vi "test_MonoOpenAndInit.vi"(6 "Delay between send and receive [ms]":i32=100, 7 "Test should pass":bool=TRUE, 8 "error in":errorcluster, 9 "tear down connection":bool=TRUE, 10 "set-up a connection":bool=TRUE, 11 "device selection":enum16{"monochromator", "CCD", "SCD"}(ring)) -> (0 "error out":errorcluster, 1 "log-file path":path)   [LabVIEW 2023]
uses:
  Classes/Mono/Monochromator.lvclass
  <vilib>/addons/_JKI Toolkits/Caraya/classes/Assert/Assert Not Error.vi
  <vilib>/addons/_JKI Toolkits/Caraya/classes/Assert/Assert Equal Value and Type_Variant.vi
  <vilib>/addons/_JKI Toolkits/Caraya/classes/Test/Test.lvclass
  <vilib>/addons/_JKI Toolkits/Caraya/classes/Assert/Assert.lvclass
  <vilib>/Hampel Software Engineering/HSE Logger/hse-logger.lvlib
  C:/Users/grju/Desktop/AbgelegteDokumente/Kunden/Horiba/horiba-labview-sdk/Source/Classes/GenericDevice/GenericDevice.lvclass
  C:/Users/grju/Desktop/AbgelegteDokumente/Kunden/Horiba/horiba-labview-sdk/Source/Classes/Mono/Monochromator.lvclass
panel:
  in  "total time out [minutes]":i32=3
  # "Connector Pane"
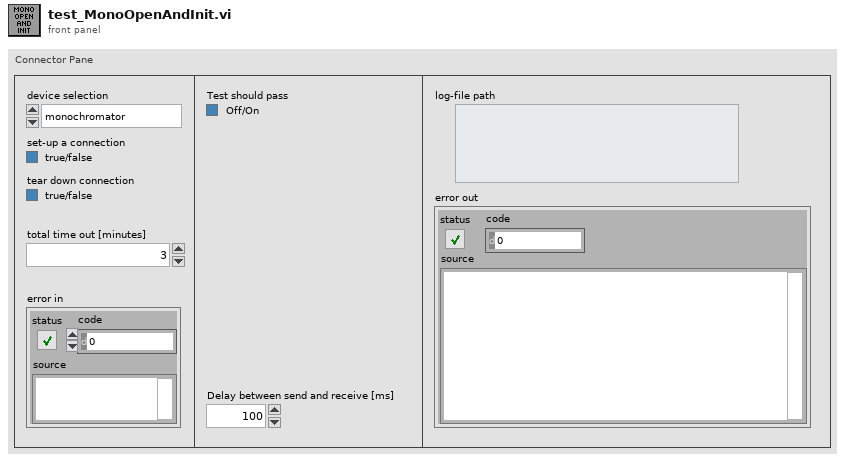
[diagram p1: front panel]
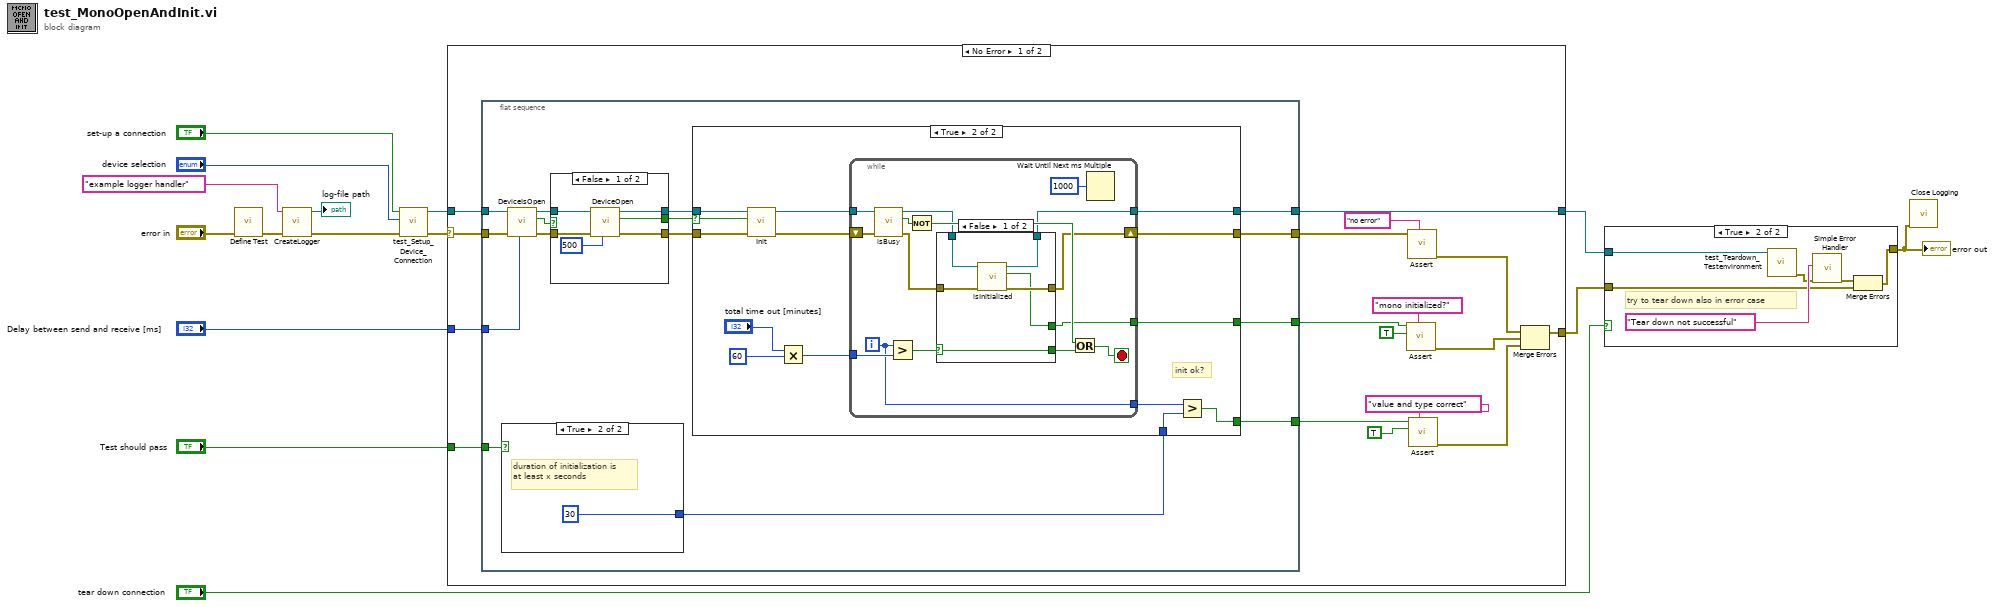
[diagram p0: block diagram]
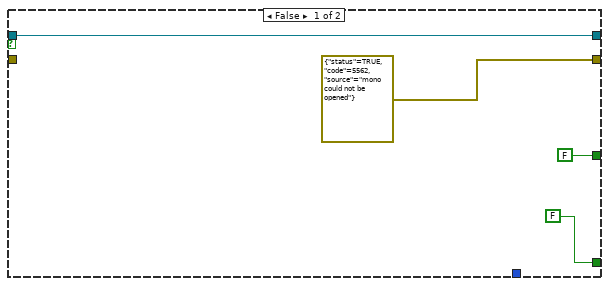
[diagram p2: hidden frame]
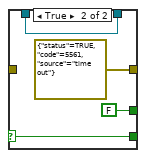
[diagram p3: hidden frame]
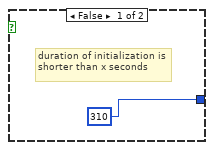
[diagram p5: hidden frame]
diagram:
  n1 = call <vilib>:"Define Test.vi"("error in (no error)"="error in") -> ("error out"=w6:errorcluster)  [unwired: 9 in, 1 out]
  n2 = call "CreateLogger.vi"("error in (no error)"=w6, "Handler Name"="example logger handler") -> ("error out"=w4:errorcluster, "log-file path"=→"log-file path":path)  [unwired: 8 in]
  n3 = call "test_Setup_Device_Connection.vi"("error in (no error)"=w4, "device selection"="device selection", "set-up a connection"="set-up a connection") -> ("error out"=w7:errorcluster, "Monochromator.lvclass"=w10:refnum<class "Monochromator.lvclass">)  [unwired: 5 in, 2 out]
  n4 = case shown="No Error" w7 {
    selector: w7 -> [w25 w103]
    tunnel: "Test should pass" -> [w30 _]
    tunnel: [w29 w102] -> w11
    tunnel: w10 -> [w28 w102]
    tunnel: [w26 w103] -> w8
    tunnel: "Delay between send and receive [ms]" -> [w24 _]
    frame No Error {
      n5 = flat-sequence {
        tunnel: w25 -> [w46]
        tunnel: w30 -> [w47]
        tunnel: [w36] -> w29
        tunnel: w28 -> [w43]
        tunnel: w24 -> [w42]
        tunnel: [w35] -> w23
        tunnel: [w34] -> w21
        tunnel: [w33] -> w16
        frame #0 {
          n6 = case shown="True" w47 {
            tunnel: [310 ("y") 30 ("y")] -> w37
            frame False {
              # "duration of initialization is shorter than x seconds"
            }
            frame True {
              # "duration of initialization is at least x seconds"
            }
          }
          n7 = call-dynamic "DeviceIsOpen.vi"("Delay between send and receive [ms]"=w42, "error in (no error)"=w46, "Monochromator in"=w43) -> ("error out"=w44:errorcluster, "device is open?"=w41:bool, "Monochromator out"=w45:refnum<class "Monochromator.lvclass">)  [unwired: 5 in, 1 out]
          n8 = case shown="False" w41 {
            selector: w41 -> [_ w97]
            tunnel: w45 -> [w96 w99]
            tunnel: [w93 w99] -> w38
            tunnel: w44 -> [w95 w98]
            tunnel: [w94 w98] -> w39
            tunnel: [w91 w97] -> w40
            frame False {
              n9 = call-dynamic "DeviceOpen.vi"("Delay between send and receive [ms]"=500, "error in (no error)"=w95, "Monochromator in"=w96) -> ("error out"=w94:errorcluster, "device is open?"=w91:bool, "Monochromator out"=w93:refnum<class "Monochromator.lvclass">)  [unwired: 5 in, 1 out]
            }
            frame True {
            }
          }
          n10 = case shown="True" w40 {
            selector: w40 -> [_ w64]
            tunnel: w39 -> [_ w63]
            tunnel: w38 -> [w49 w65]
            tunnel: [errorcluster {"status"=TRUE, "code"=5562, "source"="mono could not be opened"} ("error in 2") w56] -> w34
            tunnel: [FALSE w55] -> w35
            tunnel: w37 -> [_ w54]
            tunnel: [w49 w53] -> w36
            tunnel: [FALSE w52] -> w33
            frame False {
            }
            frame True {
              # "init ok?"
              n11 = call "Init.vi"("error in (no error)"=w63, "force"=w64, "Monochromator in"=w65) -> ("error out"=w61:errorcluster, "Monochromator out"=w62:refnum<class "Monochromator.lvclass">)  [unwired: 5 in, 2 out]
              n12 = Multiply(x="total time out [minutes]", y=60) -> (x*y=w58:i32)
              n13 = while {
                tunnel: w62 -> [w80]
                tunnel: w58 -> [w75]
                shift-right: [w70] -> w56
                shift-left: w61 -> [w79]
                tunnel: [w69] -> w57
                tunnel: [w67] -> w53
                tunnel: [w66] -> w52
                i -> [w69]
                stop <- w74 stop-if-true
                n14 = call "isBusy.vi"("error in (no error)"=w79, "Monochromator in"=w80) -> ("error out"=w71:errorcluster, "mono is busy?"=w76:bool, "Monochromator out"=w68:refnum<class "Monochromator.lvclass">)  [unwired: 7 in]
                n15 = Greater?(x=w69, y=w75) -> (0:w73:bool)
                n16 = Not(x=w76) -> (.not. x?=w77:bool)
                n17 = case shown="False" w73 {
                  selector: w73 -> [w86 w90]
                  tunnel: [w86 w90] -> w72
                  tunnel: w71 -> [w84 _]
                  tunnel: [w85 errorcluster {"status"=TRUE, "code"=5561, "source"="time out"} ("error in 2")] -> w70
                  tunnel: w68 -> [w83 w88]
                  tunnel: [w82 w88] -> w67
                  tunnel: [w81 FALSE] -> w66
                  frame False {
                    n18 = call "isInitialized.vi"("error in (no error)"=w84, "Monochromator in"=w83) -> ("error out"=w85:errorcluster, "mono is initialized?"=w81:bool, "Monochromator out"=w82:refnum<class "Monochromator.lvclass">)  [unwired: 7 in]
                  }
                  frame True {
                  }
                }
                n19 = Or(x=w77, y=w72) -> (x .or. y?=w74:bool)
                n20 = Wait Until Next ms Multiple(millisecond multiple=u32 1000) -> ()  [unwired: 1 out]
              }
              n21 = Greater?(x=w57, y=w54) -> (0:w55:bool)
            }
          }
        }
      }
      n22 = call-poly <vilib>:"Assert.vi"("Label"="mono initialized?" ("Label (VI Title)"), "Y"=TRUE, "X"=w16) -> ("error out"=w17:errorcluster)  [unwired: 7 in, 1 out]
      n23 = call-poly <vilib>:"Assert.vi"("Label"="no error" ("Label (VI Title)"), "Not Error?"=w21) -> ("error out"=w27:errorcluster)  [unwired: 8 in, 1 out]
      n24 = call-poly <vilib>:"Assert.vi"("Label"="value and type correct" ("Label (VI Title)"), "Y"=TRUE, "X"=w23) -> ("error out"=w20:errorcluster)  [unwired: 7 in, 1 out]
      n25 = Merge Errors(w27, w17, w20) -> (w26:errorcluster)
    }
    frame Error {
    }
  }
  n26 = case shown="True" "tear down connection" {
    tunnel: w11 -> [_ w109]
    tunnel: [w104 w105] -> w2
    tunnel: w8 -> [w104 w106]
    frame False {
    }
    frame True {
      # "try to tear down also in error case"
      n27 = call "test_Teardown_Testenvironment.vi"("GenericDevice.lvclass"=w109) -> ("error out"=w108:errorcluster)  [unwired: 9 in, 1 out]
      n28 = call <vilib>:"Simple Error Handler.vi"("error source (\" \")"="Tear down not successful" ("error source (\" \")"), "error in (no error)"=w108) -> ("error out"=w107:errorcluster)  [unwired: 3 in, 4 out]
      n29 = Merge Errors(w107, w106) -> (w105:errorcluster)
    }
  }
  "error out" <- w2
  n30 = call <vilib>:"Close Logging.vi"("error in"=w2) -> ()  [unwired: 10 in, 1 out]
